vi "Cannon GetSensors.vi"(1 "Cannon Global Data In":T2) -> (0 "Cannon Global Data Out":T2)   [LabVIEW 2013]
uses:
  <vilib>/Rock Robotics/WPI/Solenoid/WPI_SolenoidValue.ctl
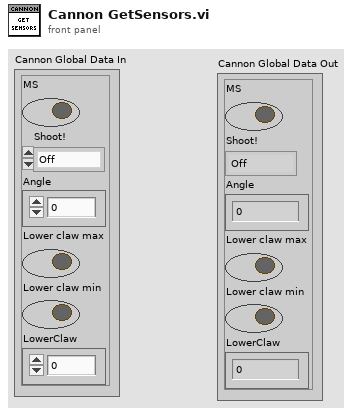
[diagram p1: front panel]
types:
  T1 = typedef "WPI_SolenoidValue.ctl" = enum16{"Off", "On", "Forward", "Reverse"}
  T2 = cluster{"MS":bool, "Shoot!":T1, "Angle":dbl, "Lower claw max":bool, "Lower claw min":bool, "LowerClaw":dbl}
  T3 = typedef "WPI_DigitalInputDevRef.ctl" = cluster{"DevStatus":errorcluster, "DIO Channel":T4, "Digital Module":T5}
  T4 = typedef "FPGA_DIOChannel.ctl" = enum8{"DIO 1", "DIO 2", "DIO 3", "DIO 4", "DIO 5", "DIO 6", "DIO 7", "DIO 8", "DIO 9", "DIO 10", "DIO 11", "DIO 12", "DIO 13", "DIO 14", "Invalid"}
  T5 = typedef "FPGA_TypedefDigitalModule.ctl" = enum16{"Digital Module 1", "Digital Module 2"}
  T6 = typedef "WPI_GyroDevRef.ctl" = cluster{"DevStatus":errorcluster, "Analog Module":T7, "Analog Channel":T8, "Offset":dbl, "Gain (VoltsPerDegree/Second)":dbl}
  T7 = typedef "FPGA_TypedefAnalogModule.ctl" = enum16{"Analog Module 1", "Analog Module 2"}
  T8 = typedef "FPGA_AIChannel.ctl" = enum8{"AI 1", "AI 2", "AI 3", "AI 4", "AI 5", "AI 6", "AI 7", "AI 8", "Invalid"}
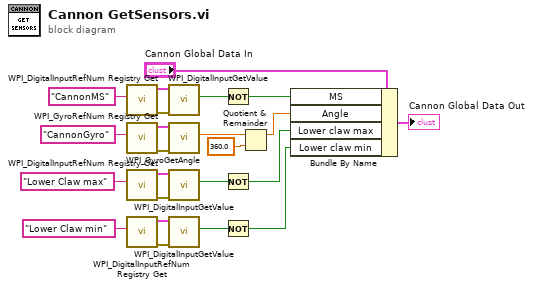
[diagram p0: block diagram]
diagram:
  n1 = call <vilib>:"WPI_DigitalInputRefNum Registry Get.vi"("refnum name"="CannonMS") -> ("error out"=w19:errorcluster, "DigitalInputDevRef"=w20:T3)  [unwired: 9 in]
  n2 = call <vilib>:"WPI_GyroRefNum Registry Get.vi"("refnum name"="CannonGyro") -> ("error out"=w8:errorcluster, "GyroDevRef"=w7:T6)  [unwired: 9 in]
  n3 = call <vilib>:"WPI_DigitalInputRefNum Registry Get.vi"("refnum name"="Lower Claw max") -> ("error out"=w13:errorcluster, "DigitalInputDevRef"=w12:T3)  [unwired: 9 in]
  n4 = call <vilib>:"WPI_DigitalInputRefNum Registry Get.vi"("refnum name"="Lower Claw min") -> ("error out"=w15:errorcluster, "DigitalInputDevRef"=w16:T3)  [unwired: 9 in]
  n5 = call <vilib>:"WPI_DigitalInputGetValue.vi"("error in (no error)"=w19, "DigitalInputDevRef"=w20) -> ("Value"=w17:bool)  [unwired: 7 in, 2 out]
  n6 = call <vilib>:"WPI_GyroGetAngle.vi"("error in (no error)"=w8, "GyroDevRef"=w7) -> ("Angle"=w6:dbl)  [unwired: 6 in, 3 out]
  n7 = call <vilib>:"WPI_DigitalInputGetValue.vi"("error in (no error)"=w13, "DigitalInputDevRef"=w12) -> ("Value"=w10:bool)  [unwired: 7 in, 2 out]
  n8 = call <vilib>:"WPI_DigitalInputGetValue.vi"("error in (no error)"=w15, "DigitalInputDevRef"=w16) -> ("Value"=w9:bool)  [unwired: 7 in, 2 out]
  n9 = Not(x=w17) -> (.not. x?=w3:bool)
  n10 = Not(x=w10) -> (.not. x?=w2:bool)
  n11 = Not(x=w9) -> (.not. x?=w1:bool)
  n12 = Quotient & Remainder(x=w6, y=360.0) -> (x-y*floor(x/y)=w21:dbl)  [unwired: 1 out]
  n13 = Bundle By Name(cluster="Cannon Global Data In", "MS"=w3, "Angle"=w21, "Lower claw max"=w2, "Lower claw min"=w1) -> (→"Cannon Global Data Out":T2)
